vi "Receive Message.vi"(6 "priority":i32, 10 "File Writer in":refnum<class "File Writer.lvclass">, 11 "Message in":refnum<class "Message.lvclass">) -> (0 "error out":errorcluster, 2 "Actor out":refnum<class "Actor.lvclass">)   [LabVIEW 2020, in "File Writer.lvlib" / "File Writer.lvclass"]
doc: "Filters for Data messages and writes these to a file. All other messages are handled normally.\nData is only written when the exception state is valid and the path is non empty."
uses:
  File Writer.lvclass
  PPL/HDH.Actor Framework.Core.Actor.lvlibp/1abvi3w/vi.lib/ActorFramework/Message/Message.lvclass
  PPL/HDH.Actor Framework.Core.Actor.lvlibp/1abvi3w/vi.lib/ActorFramework/Actor/Actor.lvclass
  C:/Current projects/WS/PPL/HDH.Actor Framework.Core.Actor.lvlibp/1abvi3w/vi.lib/ActorFramework/Actor/Actor.lvclass
  PPL/HDH.Actor Framework.Core.Publisher.lvlibp/Messages/Data Msg/Data Msg.lvclass
  File Writer.lvclass/File Writer.ctl
  PPL/HDH.Data.Generic.lvlibp/Data.lvclass
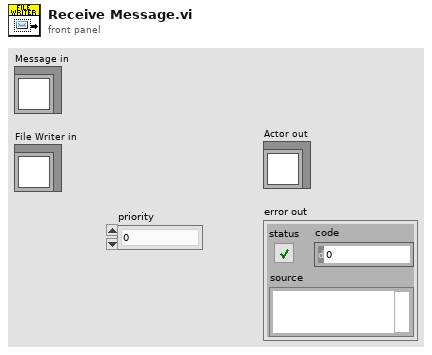
[diagram p1: front panel]
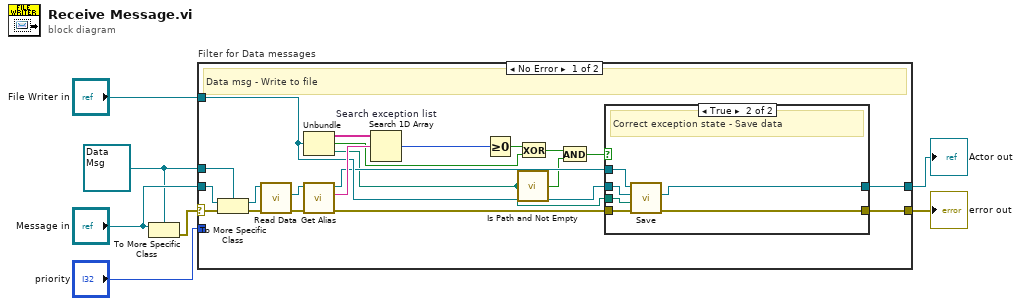
[diagram p0: block diagram]
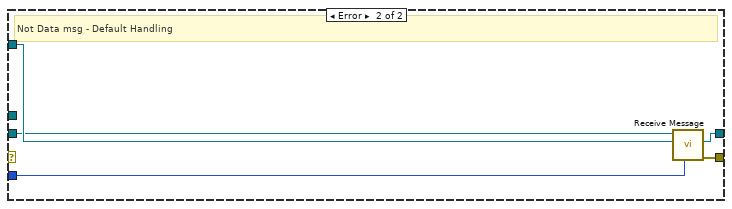
[diagram p3: hidden frame]
diagram:
  w1 = refnum<class "Data Msg.lvclass"> refnum ("HDH.Actor Framework.Core.Publisher.lvlibp:Data Msg.lvclass")
  n1 = To More Specific Class(target class=w1, reference="Message in") -> (error out=w3:errorcluster)  [unwired: 1 in, 1 out]
  n2 = case "Filter for Data messages" shown="No Error" w3 {
    selector: w3 -> [w26 _]
    tunnel: [w11 w41] -> w7
    tunnel: [w14 w40] -> w6
    tunnel: "priority" -> [_ w39]
    tunnel: "File Writer in" -> [w15 w38]
    tunnel: "Message in" -> [w28 w37]
    tunnel: w1 -> [w27 _]
    frame No Error {
      # "Data msg - Write to file"
      n3 = To More Specific Class(target class=w27, reference=w28, error in=w26) -> (specific class reference=w25:refnum<class "Data Msg.lvclass">, error out=w24:errorcluster)
      n4 = call "Read Data.vi"("error in (no error)"=w24, "Data Msg in"=w25) -> ("error out"=w20:errorcluster, "Data"=w23:refnum<class "Data.lvclass">)  [unwired: 7 in, 1 out]
      n5 = Unbundle(w15) -> (w22:string[], w17:bool, w8:path)
      n6 = call-dynamic "Get Alias.vi"("error in (no error)"=w20, "Data in"=w23) -> ("error out"=w12:errorcluster, "Alias"=w21:string, "Data out"=w13:refnum<class "Data.lvclass">)  [unwired: 7 in]
      n7 = Search 1D Array "Search exception list"(1D array=w22, element=w21) -> (index of element=w19:i32)  [unwired: 1 in]
      n8 = Greater Or Equal To 0?(x=w19) -> (x >= 0?=w18:bool)
      n9 = call <vilib>:"Is Path and Not Empty.vi"("path"=w8) -> ("Is Path and Not Empty?"=w9:bool)  [unwired: 4 in]
      n10 = Exclusive Or(1:w17, 2:w18) -> (0:w16:bool)
      n11 = And(x=w16, y=w9) -> (x .and. y?=w10:bool)
      n12 = case shown="True" w10 {
        tunnel: w15 -> [w30 w36]
        tunnel: [w30 w35] -> w14
        tunnel: w13 -> [_ w34]
        tunnel: w12 -> [w29 w33]
        tunnel: [w29 w32] -> w11
        tunnel: w8 -> [_ w31]
        frame False {
          # "Incorrect exception state - Don't save data"
        }
        frame True {
          # "Correct exception state - Save data"
          n13 = call-dynamic "Save.vi"("error in (no error)"=w33, "File Path"=w31, "File Writer in"=w36, "Data"=w34) -> ("error out"=w32:errorcluster, "Actor out"=w35:refnum<class "Actor.lvclass">)  [unwired: 6 in]
        }
      }
    }
    frame Error {
      # "Not Data msg - Default Handling"
      n14 = call-parent "Receive Message.vi"("priority"=w39, "Actor in"=w38, "Message in"=w37) -> ("error out"=w41:errorcluster, "Actor out"=w40:refnum<class "Actor.lvclass">)  [unwired: 7 in]
    }
  }
  "error out" <- w7
  "Actor out" <- w6
